vi "dummy code.vi"() -> ()   [LabVIEW 2025]
panel:
  in  "Tab Control 3":T1(tab)
  in  "Tab Control 5":enum32{""}(tab)
  in  "Tab Control 14":T2(tab)=enum."Motor Load"
  in  "Ramp MulFac":dbl=2.0
  in  "pulses LoadDiffRamp(2..10)":dbl=9.0
  in  "PulseControlRamp(diff<=3N)":dbl=5.0 min=1.0 max=1000.0 step=1.0 format="%#.1f"
  in  "SetLoadDeadband(%) Load(0-10N)":dbl=0.1 min=0.0001 max=100.0 step=0.0001 format="%#.6f"
  in  "PID gains out delay (microForce)":T3={"proportional gain (Kc)"=300.0, "integral time (Ti, min)"=0.00011, "derivative time (Td, min)"=0.0} {"derivative time (Td, min)" format="%.3f"; "integral time (Ti, min)" min=1e-05 max=100.0 step=1e-06 format="%.6f"; "proportional gain (Kc)" format="%.3f"}
  in  "Ramp":bool
  in  "Gain 2":dbl=0.016
  in  "pulses LoadDiff(2..10)":dbl=10.0
  in  "pulses LoadDiff(11..50)":dbl=40.0
  in  "PulseControl(diff<=3N)":dbl=1.0 min=1.0 max=1000.0 step=1.0 format="%#.1f"
  out "SetLoadDeadband(%)  2":dbl=1.0 min=0.001 max=100.0 step=0.001 format="%#.6f"
  in  "Dummy Run":bool
  out "Vertical load (N)":dbl format="%#.3f"
  in  "AutoTune":bool
  in  "Offset  3":dbl=1.5
  in  "apply load":bool
  in  "Enter ByPass Load":dbl
  in  "reinit 3":bool=TRUE
  in  "output range delay":cluster{"output high":dbl, "output low":dbl}={"output high"=100.0, "output low"=-100.0} {"output low" format="%.2f"; "output high" format="%.2f"}
  in  "PID gains out delay":T3={"proportional gain (Kc)"=30.0, "integral time (Ti, min)"=0.00101, "derivative time (Td, min)"=0.0} {"derivative time (Td, min)" format="%.3f"; "integral time (Ti, min)" min=1e-05 max=100.0 step=0.0001 format="%.4f"; "proportional gain (Kc)" format="%.3f"}
  in  "Bypass Load":bool
  in  "pulsesSent":dbl=200.0
  out "pulses":dbl
  out "actpid":dbl
  out "gFF Rot 7":cluster{dbl, dbl, dbl}(graph)
  in  "pulses LoadDiff(21..1000)":dbl=40.0
  in  "Delay":dbl=1.5 min=0.001 max=5.0 step=0.001 format="%#.6f"
  in  "deadband":dbl=0.2
  in  "Tab Control 26":enum32{"Page 1", "Page 2"}(tab)
  in  "ClearAll":bool
  out "Mz(Nm)":dbl[](array[numeric])
  out "My(Nm)":dbl[](array[numeric])
  out "Mx(Nm)":dbl[](array[numeric])
  in  "Save Dwell":dbl=0.015 caption="Save Dwell (sec)" min=0.0 max=5.0 step=0.001 format="%.3f"
  out "Mx":dbl[](graph)
  out "My":dbl[](graph)
  out "Mz":dbl[](graph)
  out "Fx(N)":dbl[](graph)
  out "Fy(N)":dbl[](graph)
  out "Fz(N)":dbl[](graph)
  in  "ZeroAll":bool
  in  "Acq Delay (ms)":dbl=10.0
  in  "Burst Delay (ms)":dbl=10.0
  out "model":string
  out "SN":i32
  out "FFx(N)":dbl[](array[numeric])
  in  "Sensor IP":string="192.168.1.100"
  in  "Port":i32=8080
  out "FFy(N)":dbl[](array[numeric])
  out "Load(N)":dbl[](array[numeric])
  out "AE":bool
  in  "delete Handle":bool
  in  "Create Handle":bool=TRUE
  out "ft_data":dbl[](array[numeric])=[1.0, 1.0, 1.0, 1.0, 1.0, 1.0]
  out "ft_range":dbl[](array[numeric])=[1.0, 1.0, 1.0, 1.0, 1.0, 1.0]
  in  "stop 6":bool
  out "running_flag":bool
  out "ft_udp_handle":i32
  out "get-data-return":i32
  out "get-range-return":i32
  out "zero-return":i32
  out "filter-return":i32
  out "initial-return":i32
  out "deleteHandle-result":i32
  in  "Tab Control 19":enum32{"Platform COM", "Config ", "DevInfo"}(tab)=enum."Config "
  in  "SAMPLES":dbl=100.0
  in  "Re-initilaize":bool
  in  "Filter ON/OFF":bool=TRUE
  in  "TracHomeSurgeOffsetCounts 10MM":dbl=505100.0
  in  "TracHomeSwayOffsetCounts 10MM":dbl=1432.0
  in  "Acoustic Emission:":dbl=1.0 min=0.0001 max=200.0 step=0.0001 format="%.4f"
  in  "Apply Filter (FF)":bool
  in  "Filter% 2":dbl=50.0 min=50.0 max=100.0 step=0.1 format="%.1f"
  in  "Apply Filter (Load)":bool=TRUE
  in  "Filter%":dbl=80.0 min=50.0 max=100.0 step=0.1 format="%.1f"
  in  "Sway distance (mm)":dbl=245.0
  in  "Surge distance (mm)":dbl=370.0
  in  "DataSavingLoopDelay(ms)":dbl=15.0
  in  "SAVE  2":bool
  in  "Enter Distance":bool caption="Enter Counts"
  in  "Sway Counts:":dbl=100.0 min=0.0 max=100000000.0 step=1.0 format="%.2f"
  in  "Distance (mm): 3":dbl=100.0 caption="Distance (mm):" min=0.0 max=1500.0 step=0.001 format="%.5f"
  in  "Surge Counts:":dbl=100.0 min=0.0 max=100000000.0 step=1.0 format="%.1f"
  in  "Distance (mm): 2":dbl=100.0 caption="Distance (mm):" min=0.0 max=1500.0 step=0.0001 format="%.3f"
  in  "Distance (mm):":dbl=100.0 min=0.0 max=1500.0 step=0.001 format="%.5f"
  in  "Heave Counts:":dbl=100.0 min=0.0 max=100000000.0 step=1.0
  in  "LRMHomeSurgeOffsetCounts":dbl=307197.0
  in  "LRMHomeSwayOffsetCounts":dbl=26880.0
  in  "TracHomeSurgeOffsetCounts 20MM":dbl=505100.0
  in  "TracHomeSwayOffsetCounts 20MM":dbl=1432.0
  in  "RotHomeSwayOffsetCounts":dbl=14656.0
  in  "RotHomeSurgeOffsetCounts":dbl=311465.0
  in  "Heave distance":dbl=340.0
  out "Zmm":dbl=1600.0
  out "Heave Pulses/mm":dbl=1600.0
  out "Surge Pulses/mm":dbl=1600.0
  out "Sway Pulses/mm":dbl=320.0
  in  "Heave Pitch":dbl=4.0
  in  "Surge Pitch":dbl=3.0
  in  "Sway Pitch":dbl=2.0
  in  "Heave PPR":dbl=6400.0
  in  "Surge PPR":dbl=6400.0
  in  "Sway PPR":dbl=6400.0
  # "load Aquisition off"
  # "load Aquisition On"
  # "Configuration"
  # "Limits for Heave Surge and Sway"
  # "Modules Offset Parameters"
  # "Counts-Distance Calculator"
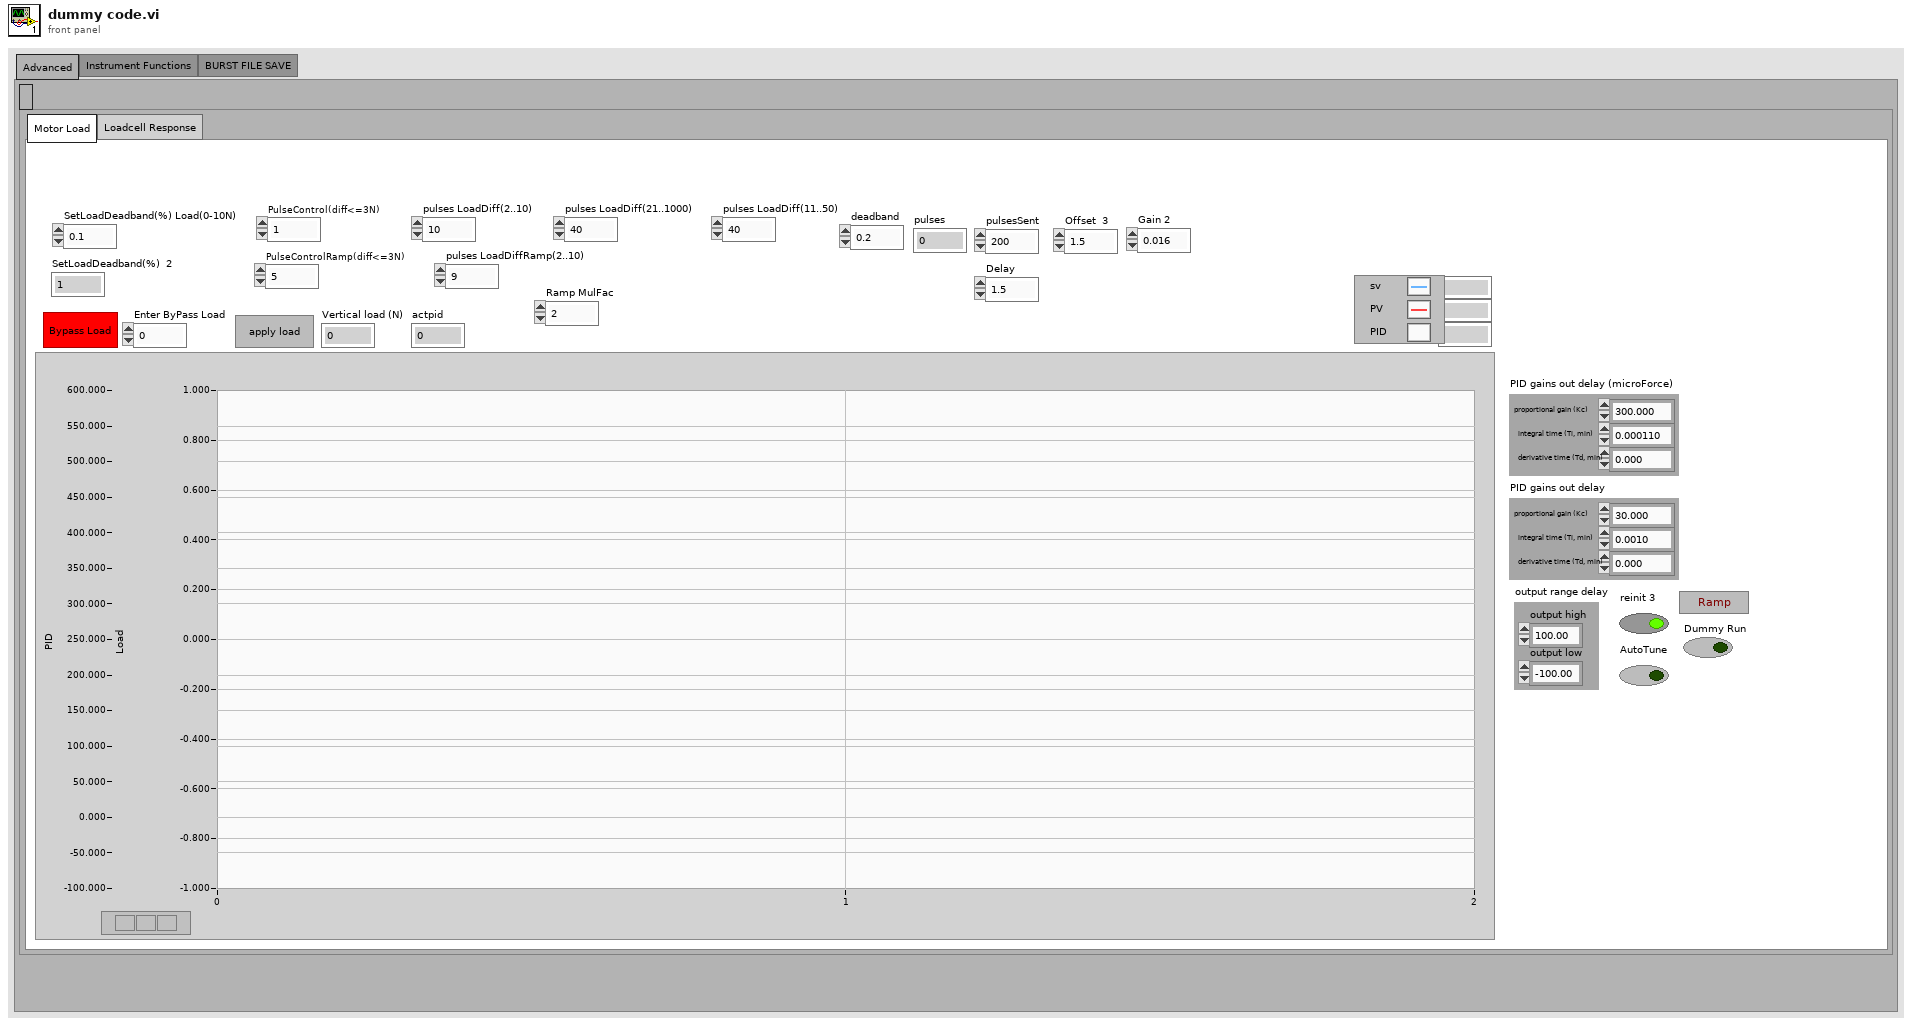
[diagram p1: front panel]
types:
  T1 = enum32{"Advanced", "Motor", "Depth_graph", "UIO Communicator", "Add to list parametrs", "Instrument Functions", "BURST FILE SAVE"}
  T2 = enum32{"LRM heating", "FBT_Heating", "Motor Load", "Loadcell Response", "Voice Load", "Step loading and speed ", "Depth"}
  T3 = cluster{"proportional gain (Kc)":dbl, "integral time (Ti, min)":dbl, "derivative time (Td, min)":dbl}
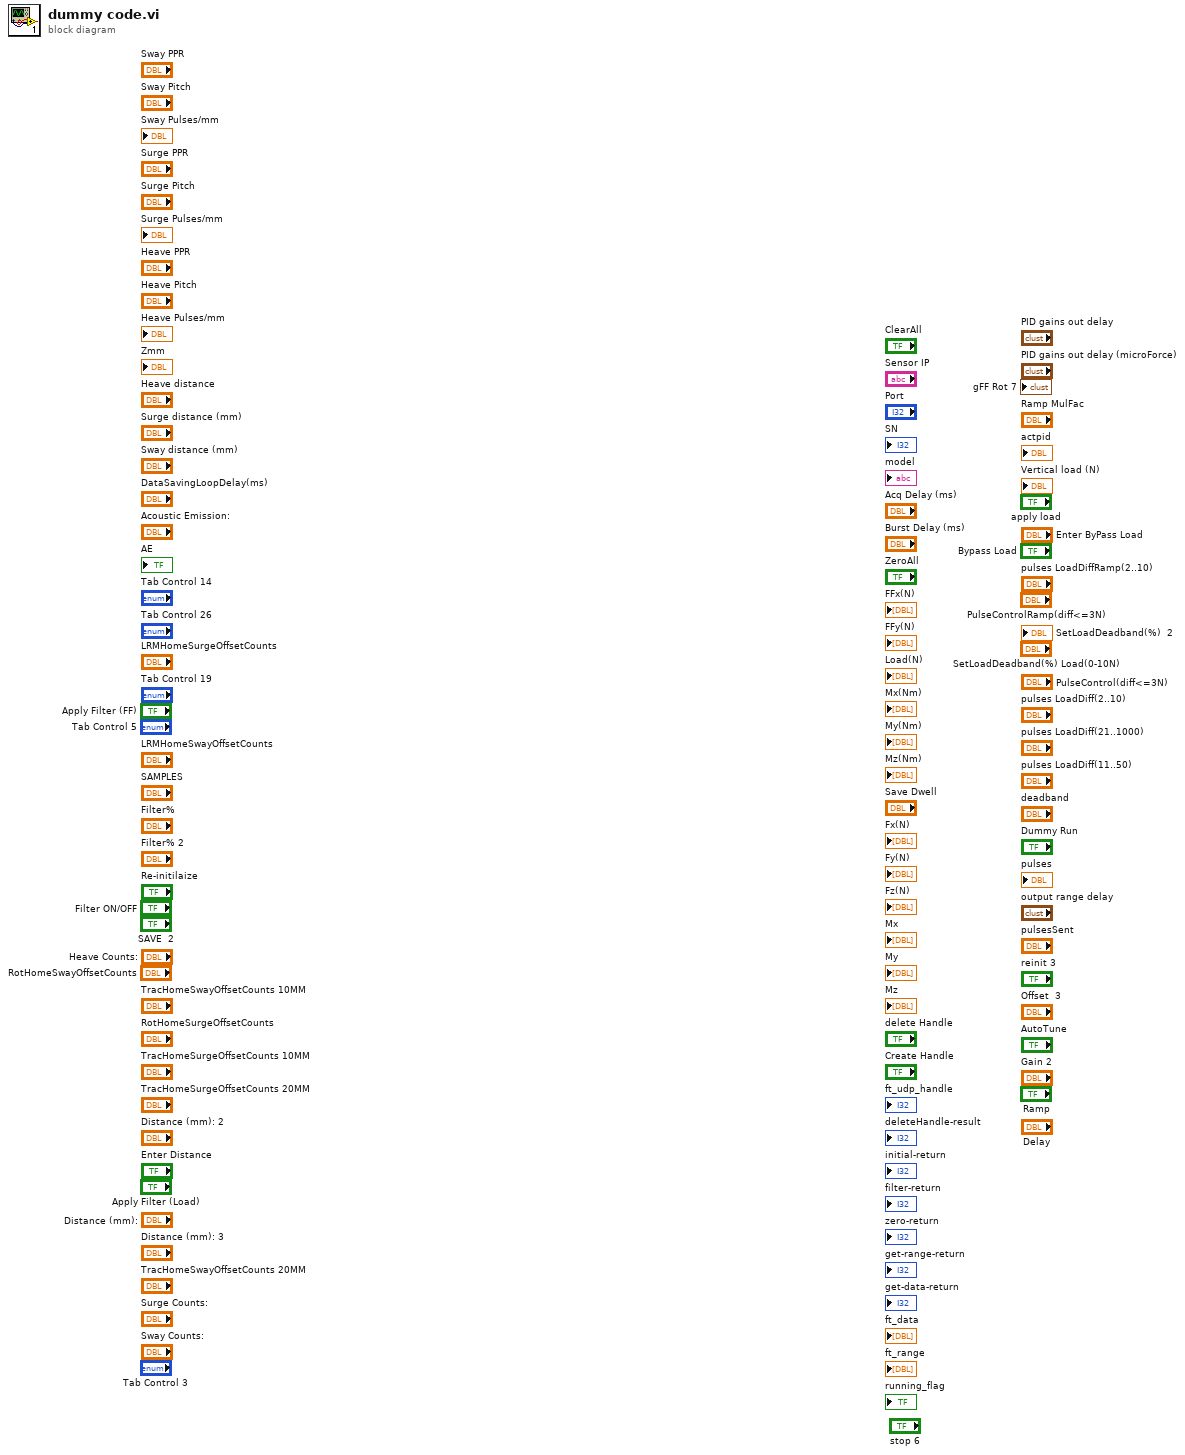
[diagram p0: block diagram]
diagram:
